vi "UI Main_V1.vi"() -> ()   [LabVIEW 2015]
uses:
  controls/UI Data.ctl
  support/Message Queue/Message Cluster.ctl
  Globals/Global - All UI Loop Stop.vi
  Globals/Global - UI Stream and Variable Connections.vi
  Globals/Global - Configuration Options.vi
  support/User Event - Stop/User Event - Stop.lvlib
  support/Message Queue/Message Queue.lvlib
panel:
  out "Current Logging State":u16(ring) items=["Logging", "Idle (Safe State)"]
  in  "Exit":bool
  out "System Status":string
  in  "Settings Tab":enum32{"UI Commands", "System Monitoring"}(tab)
  in  "Show Live Data":bool
  in  "Live Data Channel":u32 max=7 step=1
  out "Live Data":waveform(dbl)(graph)
  in  "Stop Live Data":bool
  in  "Acquire Live Data":bool
  out "Most recent manually-triggered log file":path
  in  "Force Trigger":bool
  out "Number of Data Files":u32
  out "Actual Loop Period (ticks)":u32
  out "Largest Contiguous Memory (bytes)":dbl(graph)
  out "Resource Utilization (%)":cluster{dbl, "Double":dbl, dbl}(graph)
  out "System Time":timestamp
  out "Connected?":bool
  in  "Connect to Controller":bool
  in  "Controller Address":string
  # "LabVIEW FPGA Waveform Acquisition and Logging on CompactRIO"
  # "Connection Settings"
  # "Live Data"
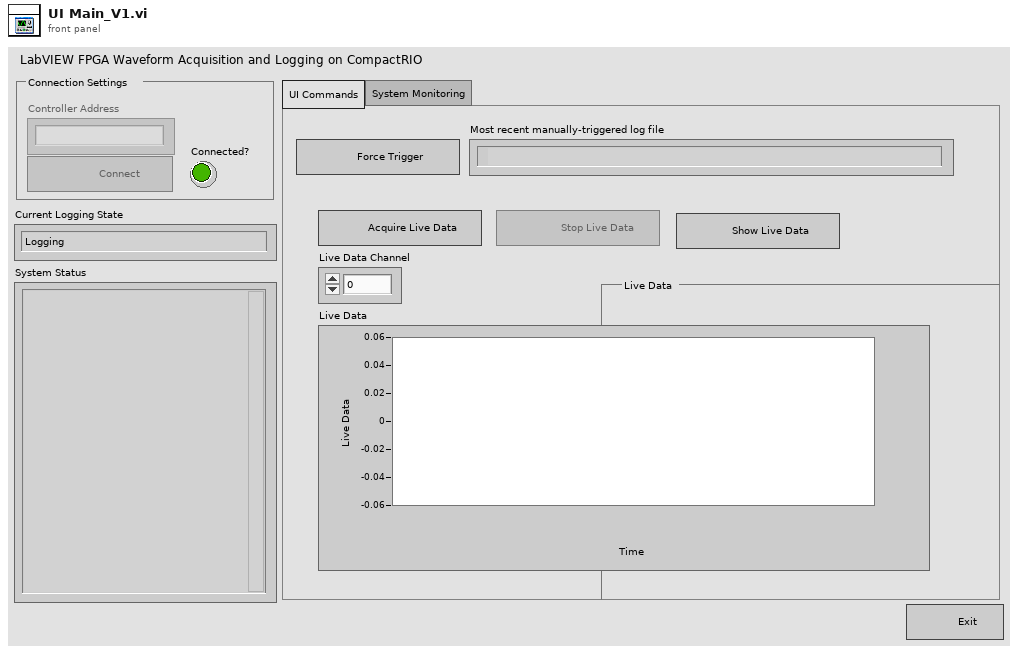
[diagram p1: front panel]
types:
  T1 = typedef "UI Data.ctl" = cluster{"Create Log File Ref":refnum<vi>, "Acquire Live Data Ref":refnum<vi>, "Stop Live Data Ref":refnum<vi>, "Show Live Data Ref":refnum<vi>}
  T2 = typedef "Message Queue.lvlib/All Host Message Queues.ctl" = cluster{"UI":refnum<queue>}
  T3 = typedef "Message Queue.lvlib/Message Cluster.ctl" = cluster{"Message":string, "Message Data":variant}
  T4 = typedef "Variable References.ctl" = cluster{"CPU Usage":refnum<k21>, "Contiguous Memory":refnum<k21>, "Actual Loop Period":refnum<k21>, "Buffer Backlog":refnum<k21>, "Drive Space":refnum<k21>, "Number of Data Files":refnum<k21>, "System Time":refnum<k21>}
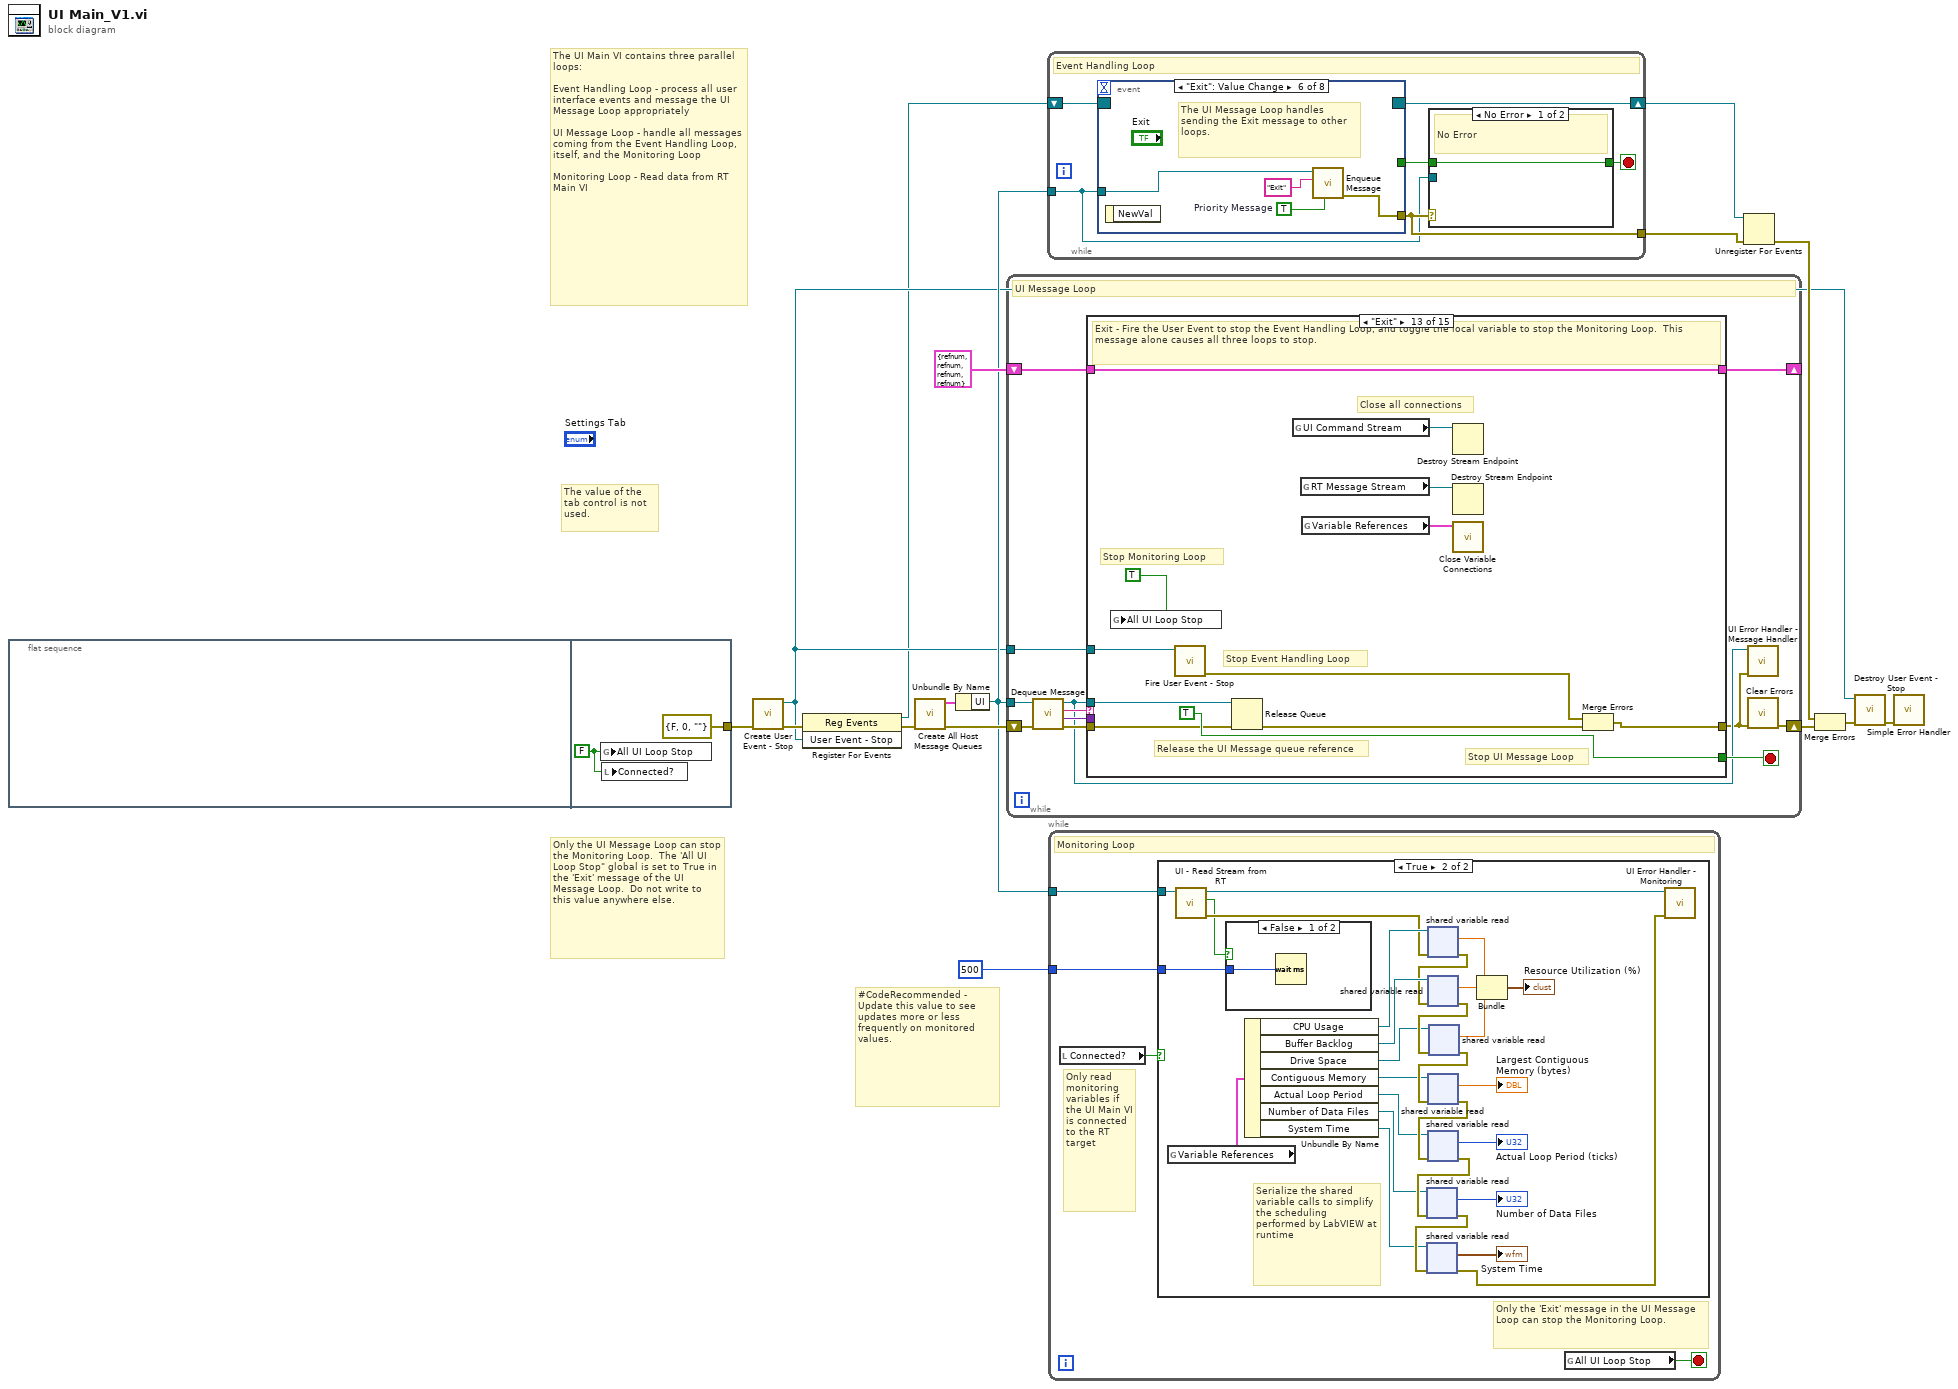
[diagram p0: block diagram]
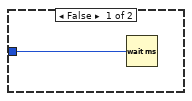
[diagram p2: hidden frame]
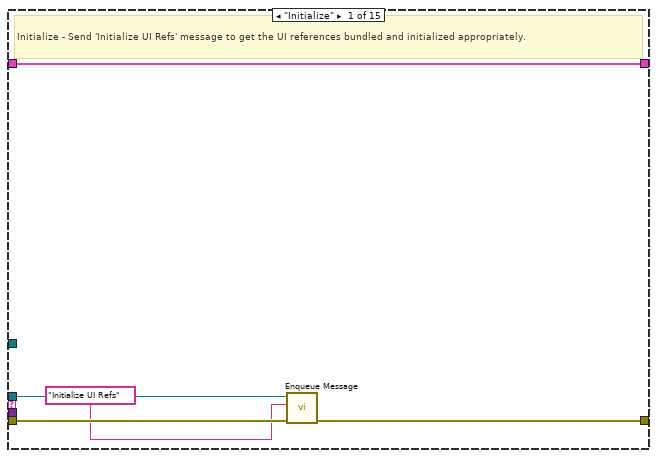
[diagram p4: hidden frame]
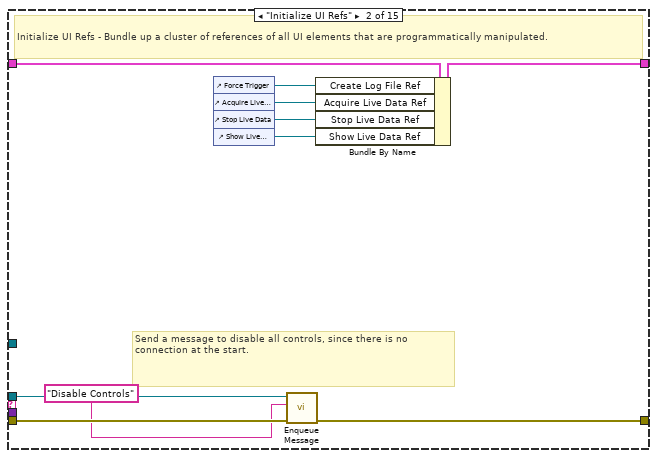
[diagram p5: hidden frame]
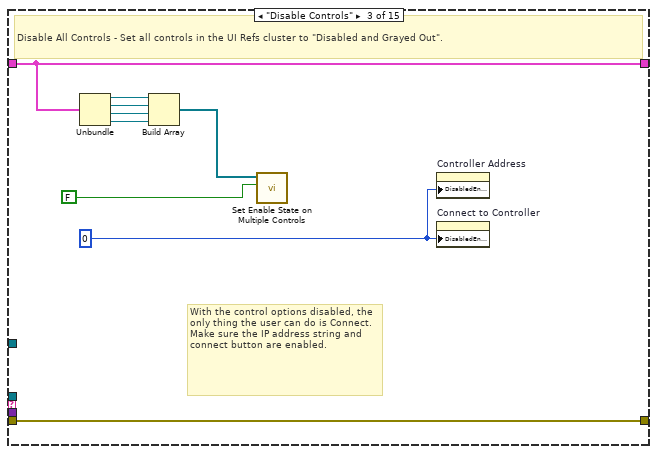
[diagram p6: hidden frame]
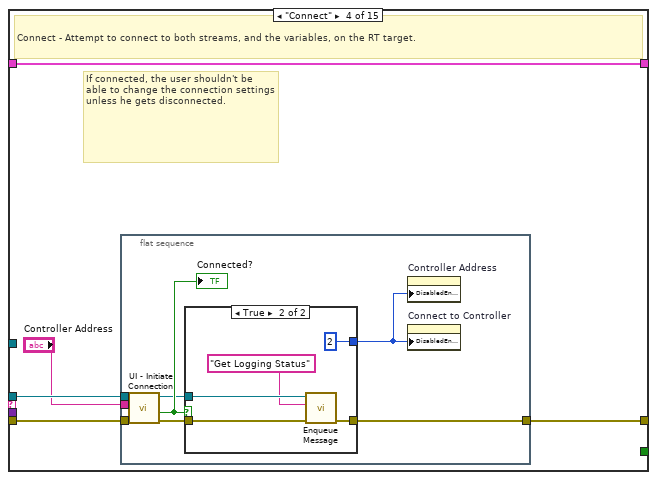
[diagram p7: hidden frame]
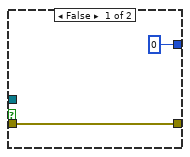
[diagram p8: hidden frame]
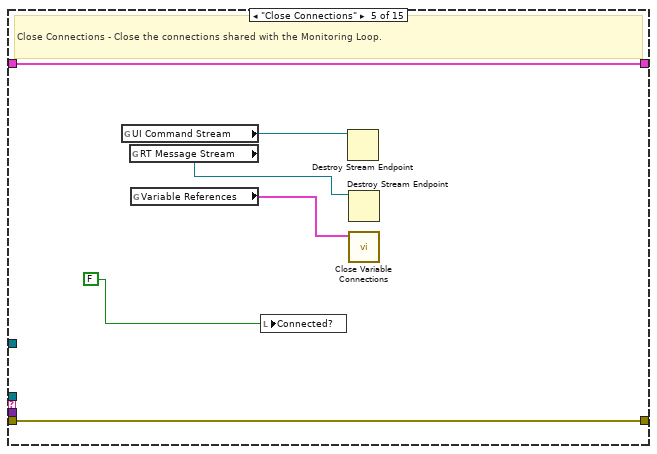
[diagram p9: hidden frame]
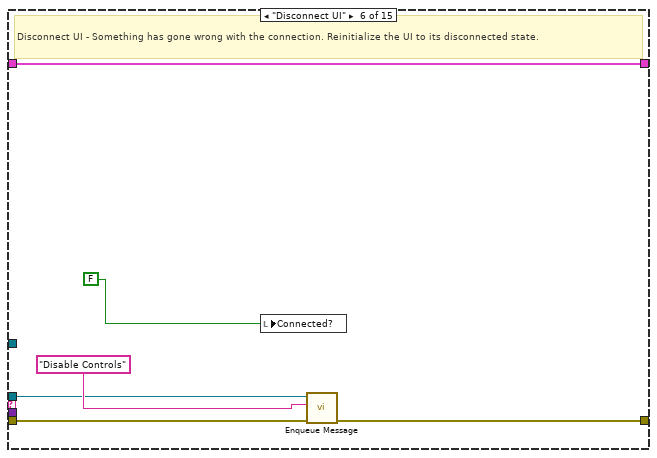
[diagram p10: hidden frame]
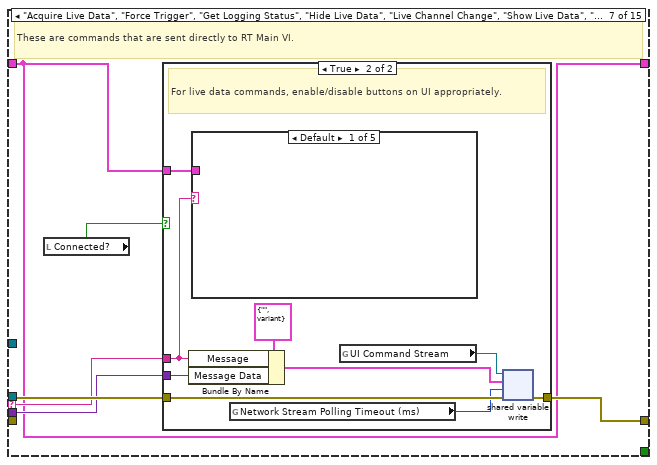
[diagram p11: hidden frame]
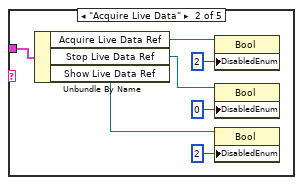
[diagram p13: hidden frame]
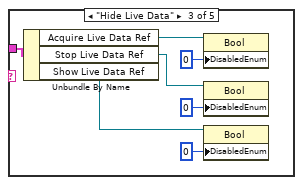
[diagram p14: hidden frame]
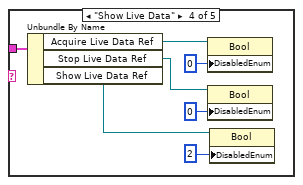
[diagram p15: hidden frame]
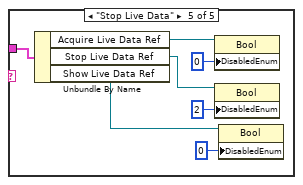
[diagram p16: hidden frame]
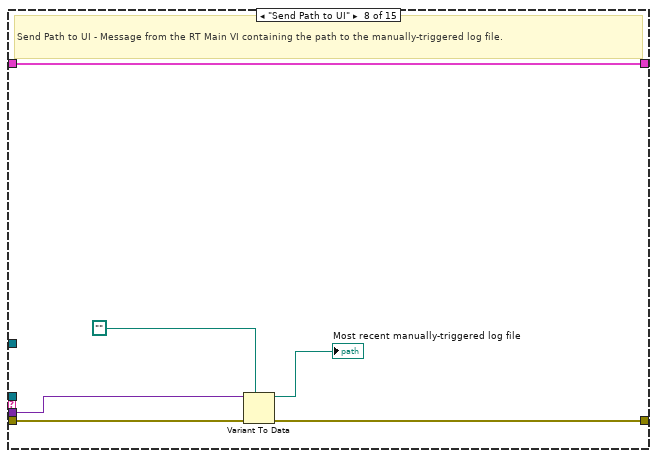
[diagram p17: hidden frame]
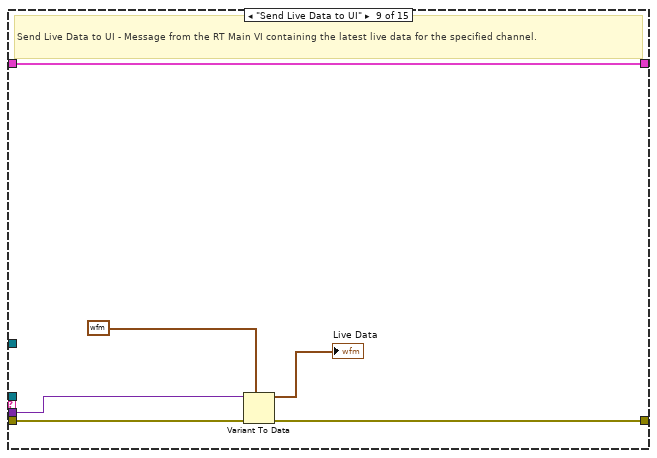
[diagram p18: hidden frame]
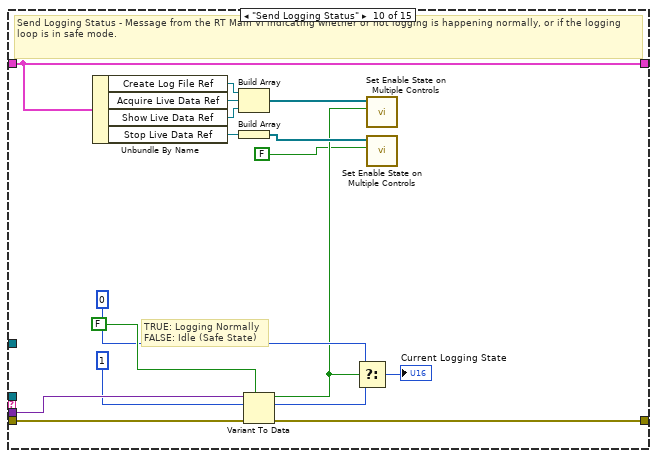
[diagram p19: hidden frame]
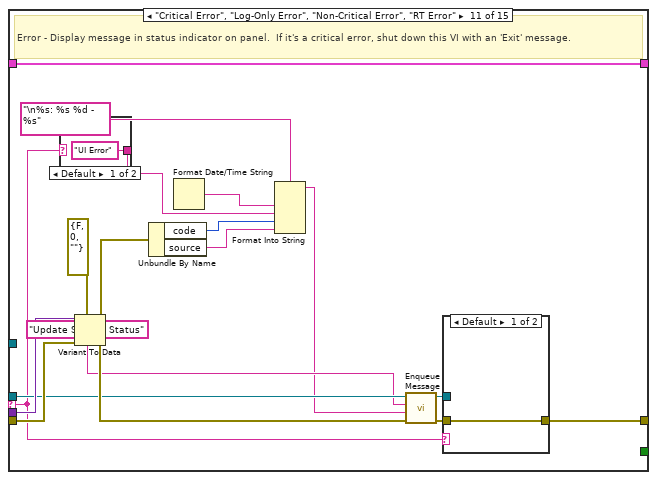
[diagram p20: hidden frame]
diagram:
  # "#CodeRecommended - Update this value to see updates more or less frequently on monitored values."
  # "The UI Main VI contains three parallel loops:\n\nEvent Handling Loop - process all user interface events and message the UI Message Loop appropriately\n\nUI Message Loop - handle all messages coming from the Event Handling Loop, itself, and the Monitoring Loop\n\nMonitoring Loop - Read data from RT Main VI"
  # "The value of the tab control is not used."
  # "Only the UI Message Loop can stop the Monitoring Loop.  The 'All UI Loop Stop\" global is set to True in the 'Exit' message of the UI Message Loop.  Do not write to this value anywhere else."
  n1 = flat-sequence {
    tunnel: [errorcluster {"status"=FALSE, "code"=0, "source"=""} ("error in (no error)")] -> w6
    frame #0 {
    }
    frame #1 {
      w17 = FALSE
      n2 = global write "Global - All UI Loop Stop.vi" "All UI Loop Stop"(w17) -> ()
      n3 = local write "Connected?"(w17) -> ()
    }
  }
  n4 = call "Create User Event - Stop.vi"("error in (no error)"=w6) -> ("error out"=w4:errorcluster, "User Event - Stop"=w2:refnum<user-event>)  [unwired: 9 in]
  n5 = register-events(error in=w4, w2) -> (reference out=w1:refnum<event-registration>, error out=w3:errorcluster)  [unwired: 1 in]
  n6 = call "Create All Host Message Queues.vi"("error in (no error)"=w3) -> ("error out"=w12:errorcluster, "Message Queues out"=w13:T2)  [unwired: 9 in]
  n7 = Unbundle By Name(w13) -> ("UI"=w7:refnum<queue>)
  n8 = while {
    tunnel: w7 -> [w24]
    tunnel: w2 -> [w29]
    shift-right: [w19] -> w16
    shift-left: w12 -> [w28]
    shift-right: [w22] -> _
    shift-left: T1 {"Create Log File Ref"=refnum, "Acquire Live Data Ref"=refnum, "Stop Live Data Ref"=refnum, "Show Live Data Ref"=refnum} ("Measurement UI Controls") -> [w23]
    stop <- w30 stop-if-true
    # "UI Message Loop"
    n9 = call "Dequeue Message.vi"("error in (no error)"=w28, "Message Queue"=w24) -> ("error out"=w27:errorcluster, "Message Data"=w25:variant, "Message"=w26:string, "dup Message Queue"=w21:refnum<queue>)  [unwired: 6 in]
    n10 = case "Message Cases" shown="\"Exit\"" w26 {
      selector: w26 -> [_ _ _ _ _ _ w89 _ _ _ w160 _ _ _ w221]
      tunnel: w21 -> [w32 w41 _ w58 _ w82 _ _ _ _ w164 _ w206 _ _]
      tunnel: w27 -> [w34 w45 w54 w59 w80 w84 w92 w136 w142 w158 w174 w195 w211 w216 _]
      tunnel: [w33 w42 w54 w56 w80 w83 w91 w134 w140 w157 w175 w193 w212 w215 w219] -> w20
      tunnel: [_ _ _ _ _ _ _ _ _ _ _ _ TRUE _ _] -> w30
      tunnel: w25 -> [_ _ _ _ _ _ w90 w133 w139 w156 w172 w192 _ _ _]
      tunnel: w29 -> [_ _ _ _ _ _ _ _ _ _ _ _ w210 _ _]
      tunnel: w23 -> [w35 w44 w53 w57 w79 w86 w88 w135 w141 w151 w176 w194 w208 w214 w217]
      tunnel: [w35 w43 w53 w57 w79 w86 w88 w135 w141 w151 w176 w194 w208 w214 w217] -> w22
      frame "Initialize" {
        # "Initialize - Send 'Initialize UI Refs' message to get the UI references bundled and initialized appropriately."
        n11 = call "Enqueue Message.vi"("error in (no error)"=w34, "Message"="Initialize UI Refs", "Message Queue"=w32) -> ("error out"=w33:errorcluster)  [unwired: 7 in, 1 out]
      }
      frame "Initialize UI Refs" {
        # "Send a message to disable all controls, since there is no connection at the start."
        # "Initialize UI Refs - Bundle up a cluster of references of all UI elements that are programmatically manipulated."
        n12 = control-ref of="Force Trigger"() -> (w39:refnum<vi>)
        n13 = control-ref of="Acquire Live Data"() -> (w38:refnum<vi>)
        n14 = control-ref of="Stop Live Data"() -> (w37:refnum<vi>)
        n15 = control-ref of="Show Live Data"() -> (w36:refnum<vi>)
        n16 = call "Enqueue Message.vi"("error in (no error)"=w45, "Message"="Disable Controls", "Message Queue"=w41) -> ("error out"=w42:errorcluster)  [unwired: 7 in, 1 out]
        n17 = Bundle By Name(cluster=w44, "Create Log File Ref"=w39, "Acquire Live Data Ref"=w38, "Stop Live Data Ref"=w37, "Show Live Data Ref"=w36) -> (w43:T1)
      }
      frame "Disable Controls" {
        w49 = 0
        # "With the control options disabled, the only thing the user can do is Connect. Make sure the IP address string and connect button are enabled."
        # "Disable All Controls - Set all controls in the UI Refs cluster to \"Disabled and Grayed Out\"."
        n18 = Unbundle(w53) -> ("Create Log File Ref"=w52:refnum<vi>, "Acquire Live Data Ref"=w48:refnum<vi>, "Stop Live Data Ref"=w47:refnum<vi>, "Show Live Data Ref"=w46:refnum<vi>)
        n19 = Build Array(w52, w48, w47, w46) -> (w51:refnum<vi>[])
        n20 = call "Set Enable State on Multiple Controls.vi"("Enable?"=FALSE, "Controls"=w51) -> ()  [unwired: 10 in]
        n21 = property on="Controller Address" class="Str"("DisabledEnum"=w49) -> ()  [unwired: 2 in, 2 out]
        n22 = property on="Connect to Controller" class="Bool"("DisabledEnum"=w49) -> ()  [unwired: 2 in, 2 out]
      }
      frame "Connect" {
        # "If connected, the user shouldn't be able to change the connection settings unless he gets disconnected."
        # "Connect - Attempt to connect to both streams, and the variables, on the RT target."
        n23 = flat-sequence {
          tunnel: [w62] -> w56
          tunnel: w59 -> [w67]
          tunnel: w58 -> [w66]
          tunnel: "Controller Address" -> [w65]
          frame #0 {
            n24 = call "UI - Initiate Connection.vi"("error in (no error)"=w67, "Controller Address"=w65, "Message Queue"=w66) -> ("error out"=w64:errorcluster, "Connected?"=w63:bool, "dup Message Queue"=w61:refnum<queue>)  [unwired: 6 in]
            "Connected?" <- w63
            n25 = case shown="True" w63 {
              tunnel: w64 -> [w69 w73]
              tunnel: [w69 w74] -> w62
              tunnel: w61 -> [_ w72]
              tunnel: [0 2] -> w60
              frame False {
              }
              frame True {
                n26 = call "Enqueue Message.vi"("error in (no error)"=w73, "Message"="Get Logging Status", "Message Queue"=w72) -> ("error out"=w74:errorcluster)  [unwired: 7 in, 1 out]
              }
            }
            n27 = property on="Controller Address" class="Str"("DisabledEnum"=w60) -> ()  [unwired: 2 in, 2 out]
            n28 = property on="Connect to Controller" class="Bool"("DisabledEnum"=w60) -> ()  [unwired: 2 in, 2 out]
          }
        }
      }
      frame "Close Connections" {
        # "Close Connections - Close the connections shared with the Monitoring Loop."
        n29 = global read "Global - UI Stream and Variable Connections.vi" "UI Command Stream"() -> (w78:refnum<k21>)
        n30 = global read "Global - UI Stream and Variable Connections.vi" "RT Message Stream"() -> (w77:refnum<k21>)
        n31 = global read "Global - UI Stream and Variable Connections.vi" "Variable References"() -> (w76:T4)
        n32 = local write "Connected?"(FALSE ("Connected?")) -> ()
        n33 = Destroy Stream Endpoint(11:w78) -> ()  [unwired: 1 in, 1 out]
        n34 = Destroy Stream Endpoint(11:w77) -> ()  [unwired: 1 in, 1 out]
        n35 = call "Close Variable Connections.vi"("Variable References"=w76) -> ()  [unwired: 11 in]
      }
      frame "Disconnect UI" {
        # "Disconnect UI - Something has gone wrong with the connection. Reinitialize the UI to its disconnected state."
        n36 = local write "Connected?"(FALSE ("Connected?")) -> ()
        n37 = call "Enqueue Message.vi"("error in (no error)"=w84, "Message"="Disable Controls", "Message Queue"=w82) -> ("error out"=w83:errorcluster)  [unwired: 7 in, 1 out]
      }
      frame "Acquire Live Data", "Force Trigger", "Get Logging Status", "Hide Live Data", "Live Channel Change", "Show Live Data", "Stop Live Data" {
        # "These are commands that are sent directly to RT Main VI."
        n38 = local read "Connected?"() -> (w87:bool)
        n39 = case shown="True" w87 {
          tunnel: w92 -> [w93 w102]
          tunnel: [w93 w101] -> w91
          tunnel: w90 -> [_ w96]
          tunnel: w89 -> [_ w94]
          tunnel: w88 -> [_ w95]
          frame False {
            # "Don't bother trying to send a message to the RT system if UI Main VI isn't even connected"
          }
          frame True {
            # "For live data commands, enable/disable buttons on UI appropriately."
            n40 = Bundle By Name(cluster=T3 {"Message"="", "Message Data"=variant} ("Message Cluster"), "Message"=w94, "Message Data"=w96) -> (w97:T3)
            n41 = case shown="Default" w94 {
              tunnel: w95 -> [_ w109 w110 w119 w130]
              frame Default {
              }
              frame "Acquire Live Data" {
                n42 = Unbundle By Name(w109) -> ("Acquire Live Data Ref"=w108:refnum<vi>, "Stop Live Data Ref"=w107:refnum<vi>, "Show Live Data Ref"=w103:refnum<vi>)
                n43 = property class="Bool"(reference=w108, "DisabledEnum"=u8 2) -> ()  [unwired: 1 in, 2 out]
                n44 = property class="Bool"(reference=w107, "DisabledEnum"=u8 0) -> ()  [unwired: 1 in, 2 out]
                n45 = property class="Bool"(reference=w103, "DisabledEnum"=u8 2) -> ()  [unwired: 1 in, 2 out]
              }
              frame "Hide Live Data" {
                n46 = Unbundle By Name(w110) -> ("Acquire Live Data Ref"=w116:refnum<vi>, "Stop Live Data Ref"=w115:refnum<vi>, "Show Live Data Ref"=w111:refnum<vi>)
                n47 = property class="Bool"(reference=w116, "DisabledEnum"=u8 0) -> ()  [unwired: 1 in, 2 out]
                n48 = property class="Bool"(reference=w115, "DisabledEnum"=u8 0) -> ()  [unwired: 1 in, 2 out]
                n49 = property class="Bool"(reference=w111, "DisabledEnum"=u8 0) -> ()  [unwired: 1 in, 2 out]
              }
              frame "Show Live Data" {
                n50 = Unbundle By Name(w119) -> ("Acquire Live Data Ref"=w123:refnum<vi>, "Stop Live Data Ref"=w122:refnum<vi>, "Show Live Data Ref"=w118:refnum<vi>)
                n51 = property class="Bool"(reference=w123, "DisabledEnum"=u8 0) -> ()  [unwired: 1 in, 2 out]
                n52 = property class="Bool"(reference=w122, "DisabledEnum"=u8 0) -> ()  [unwired: 1 in, 2 out]
                n53 = property class="Bool"(reference=w118, "DisabledEnum"=u8 2) -> ()  [unwired: 1 in, 2 out]
              }
              frame "Stop Live Data" {
                n54 = Unbundle By Name(w130) -> ("Acquire Live Data Ref"=w129:refnum<vi>, "Stop Live Data Ref"=w128:refnum<vi>, "Show Live Data Ref"=w124:refnum<vi>)
                n55 = property class="Bool"(reference=w129, "DisabledEnum"=u8 0) -> ()  [unwired: 1 in, 2 out]
                n56 = property class="Bool"(reference=w128, "DisabledEnum"=u8 2) -> ()  [unwired: 1 in, 2 out]
                n57 = property class="Bool"(reference=w124, "DisabledEnum"=u8 0) -> ()  [unwired: 1 in, 2 out]
              }
            }
            n58 = global read "Global - Configuration Options.vi" "Network Stream Polling Timeout (ms)"() -> (w99:i32)
            n59 = global read "Global - UI Stream and Variable Connections.vi" "UI Command Stream"() -> (w100:refnum<k21>)
            n60 = shared-variable-write(w100, w102, w97, w99) -> (w101:errorcluster)  [unwired: 2 out]
          }
        }
      }
      frame "Send Path to UI" {
        # "Send Path to UI - Message from the RT Main VI containing the path to the manually-triggered log file."
        n61 = Variant To Data(error in=w136, type=path "", Variant=w133) -> (data=→"Most recent manually-triggered log file":path, error out=w134:errorcluster)
      }
      frame "Send Live Data to UI" {
        # "Send Live Data to UI - Message from the RT Main VI containing the latest live data for the specified channel."
        n62 = Variant To Data(error in=w142, type=waveform(dbl) {"t0"=timestamp(0 s since 1904-01-01), "dt"=1.0, "Y"=[]}, Variant=w139) -> (data=→"Live Data":waveform(dbl), error out=w140:errorcluster)
      }
      frame "Send Logging Status" {
        # "TRUE: Logging Normally\nFALSE: Idle (Safe State)"
        # "Send Logging Status - Message from the RT Main VI indicating whether or not logging is happening normally, or if the logging loop is in safe mode."
        n63 = Unbundle By Name(w151) -> ("Create Log File Ref"=w150:refnum<vi>, "Acquire Live Data Ref"=w149:refnum<vi>, "Show Live Data Ref"=w144:refnum<vi>, "Stop Live Data Ref"=w143:refnum<vi>)
        n64 = Build Array(w150, w149, w144) -> (w148:refnum<vi>[])
        n65 = Build Array(w143) -> (w147:refnum<vi>[])
        n66 = Variant To Data(error in=w158, type=FALSE, Variant=w156) -> (data=w146:bool, error out=w157:errorcluster)
        n67 = Select(t=u16 0, s=w146, f=u16 1) -> (s? t:f=→"Current Logging State":u16)
        n68 = call "Set Enable State on Multiple Controls.vi"("Enable?"=w146, "Controls"=w148) -> ()  [unwired: 10 in]
        n69 = call "Set Enable State on Multiple Controls.vi"("Enable?"=FALSE, "Controls"=w147) -> ()  [unwired: 10 in]
      }
      frame "Critical Error", "Log-Only Error", "Non-Critical Error", "RT Error" {
        # "Error - Display message in status indicator on panel.  If it's a critical error, shut down this VI with an 'Exit' message."
        n70 = case shown="Default" w160 {
          selector: w160 -> [_ w183]
          tunnel: ["UI Error" w183] -> w159
          frame Default {
          }
          frame "RT Error" {
          }
        }
        n71 = Variant To Data(error in=w174, type=errorcluster {"status"=FALSE, "code"=0, "source"=""} ("error constant"), Variant=w172) -> (data=w167:errorcluster, error out=w173:errorcluster)
        n72 = Unbundle By Name(w167) -> ("code"=w166:i32, "source"=w170:string)
        n73 = Format Date/Time String() -> (date/time string=w169:string)  [unwired: 3 in]
        n74 = Format Into String(format string="\n%s: %s %d - %s", w169, w159, w166, w170) -> (resulting string=w161:string)  [unwired: 2 in, 1 out]
        n75 = call "Enqueue Message.vi"("error in (no error)"=w173, "Message Data"=w161, "Message"="Update System Status", "Message Queue"=w164) -> ("error out"=w165:errorcluster, "dup Message Queue"=w163:refnum<queue>)  [unwired: 6 in]
        n76 = case shown="Default" w160 {
          tunnel: w165 -> [w177 w181]
          tunnel: w163 -> [_ w179]
          tunnel: [w177 w180] -> w175
          frame Default {
          }
          frame "Critical Error" {
            n77 = call "Enqueue Message.vi"("error in (no error)"=w181, "Message"="Exit", "Message Queue"=w179) -> ("error out"=w180:errorcluster)  [unwired: 7 in, 1 out]
          }
        }
      }
      frame "Update System Status" {
        # "#CodeRecommended - The code below ensures that the System Status string value does not become too large.  It uses the same maximum size as the RT error log to determine whether or not to remove the last half of the log string. Change this logic if you wish to maintain more/less of the information in the System Status string."
        # "Update System Status - Add a new string to the beginning of the System Status string on the UI."
        n78 = Variant To Data(error in=w195, type="", Variant=w192) -> (data=w189:string, error out=w193:errorcluster)
        n79 = global read "Global - Configuration Options.vi" "Error Log Max Size (bytes)"() -> (w185:i64)
        n80 = local read "System Status"() -> (w187:string)
        n81 = String Length(string=w187) -> (length=w188:i32)
        n82 = Greater?(x=w188, y=w185) -> (0:w186:bool)
        n83 = case shown="True" w186 {
          tunnel: w187 -> [w196 w200]
          tunnel: w185 -> [_ w199]
          tunnel: [w196 w201] -> w184
          frame False {
          }
          frame True {
            n84 = Divide(x=w199, y=i64 2) -> (x/y=w198:dbl)
            n85 = String Subset(string=w200, length (rest)=w198) -> (substring=w201:string)  [unwired: 1 in]
          }
        }
        n86 = Concatenate Strings(w189, w184) -> (→"System Status":string)
      }
      frame "Exit" {
        # "Close all connections"
        # "Stop Monitoring Loop"
        # "Stop Event Handling Loop"
        # "Release the UI Message queue reference"
        # "Stop UI Message Loop"
        # "Exit - Fire the User Event to stop the Event Handling Loop, and toggle the local variable to stop the Monitoring Loop.  This message alone causes all three loops to stop."
        n87 = global write "Global - All UI Loop Stop.vi" "All UI Loop Stop"(TRUE ("Stop Monitoring Loop")) -> ()
        n88 = call "Fire User Event - Stop.vi"("User Event - Stop"=w210) -> ("error out"=w209:errorcluster)  [unwired: 10 in]
        n89 = Release Queue(queue=w206, error in (no error)=w211) -> (error out=w207:errorcluster)  [unwired: 1 in, 2 out]
        n90 = global read "Global - UI Stream and Variable Connections.vi" "UI Command Stream"() -> (w204:refnum<k21>)
        n91 = global read "Global - UI Stream and Variable Connections.vi" "RT Message Stream"() -> (w203:refnum<k21>)
        n92 = global read "Global - UI Stream and Variable Connections.vi" "Variable References"() -> (w202:T4)
        n93 = Destroy Stream Endpoint(11:w204) -> ()  [unwired: 1 in, 1 out]
        n94 = Destroy Stream Endpoint(11:w203) -> ()  [unwired: 1 in, 1 out]
        n95 = call "Close Variable Connections.vi"("Variable References"=w202) -> ()  [unwired: 11 in]
        n96 = Merge Errors(w209, w207) -> (w212:errorcluster)
      }
      frame "---Copy This Frame---" {
        # "Duplicate this frame when creating new messages.  Change this comment in the duplicated frame to describe this message."
        n97 = Merge Errors(w216) -> (w215:errorcluster)
      }
      frame Default {
        # "'Default' case only runs if there is a message that isn't defined in any of the other cases.  Output a programming error."
        n98 = Format Into String(format string="The invalid message string \"%s\" was received in the Message Handling Loop." ("Invalid Message Loop Message"), w221) -> (resulting string=w218:string)  [unwired: 2 in, 1 out]
        n99 = call <vilib>:"Error Cluster From Error Code.vi"("error message (\"\")"=w218, "error code (0)"=1) -> ("error out"=w219:errorcluster)  [unwired: 7 in]
      }
    }
    n100 = call "UI Error Handler - Message Handler.vi"("error in (no error)"=w20, "Message Queue"=w21) -> ()  [unwired: 9 in, 1 out]
    n101 = call <vilib>:"Clear Errors.vi"("error in (no error)"=w20) -> ("error out"=w19:errorcluster)  [unwired: 5 in, 1 out]
  }
  n102 = while {
    tunnel: w7 -> [w224]
    tunnel: [w226] -> w15
    shift-right: [w223] -> w10
    shift-left: w1 -> [w225]
    stop <- w227 stop-if-true
    # "Event Handling Loop"
    n103 = event shown="[5] \"Exit\": Value Change" {
      selector: w225 -> [_ _ _ _ _ _ _ _]
      dyn-events: [_ _ _ _ _ _ _ _] -> w223
      timeout: _ -> [_ _ _ _ _ _ _ _]
      tunnel: [_ _ _ _ _ _ TRUE ("Discard?") _] -> w228
      tunnel: w224 -> [w234 w237 w240 w243 w247 w250 _ w260]
      tunnel: [w236 w239 w242 w245 w249 w253 _ w259] -> w226
      event "Connect to Controller": Value Change {
        n104 = event-data() -> ()  [unwired: 1 in, 1 out]
        n105 = call "Enqueue Message.vi"("Message"="Connect", "Message Queue"=w234) -> ("error out"=w236:errorcluster)  [unwired: 8 in, 1 out]
      }
      event "Force Trigger": Value Change {
        n106 = event-data() -> ()  [unwired: 1 in, 1 out]
        n107 = call "Enqueue Message.vi"("Message"="Force Trigger", "Message Queue"=w237) -> ("error out"=w239:errorcluster)  [unwired: 8 in, 1 out]
      }
      event "Acquire Live Data": Value Change {
        n108 = event-data() -> ()  [unwired: 1 in, 1 out]
        n109 = call "Enqueue Message.vi"("Message"="Acquire Live Data", "Message Queue"=w240) -> ("error out"=w242:errorcluster)  [unwired: 8 in, 1 out]
      }
      event "Stop Live Data": Value Change {
        n110 = event-data() -> ()  [unwired: 1 in, 1 out]
        n111 = call "Enqueue Message.vi"("Message"="Stop Live Data", "Message Queue"=w243) -> ("error out"=w245:errorcluster)  [unwired: 8 in, 1 out]
      }
      event "Live Data Channel": Value Change {
        n112 = event-data() -> ()  [unwired: 1 in, 1 out]
        n113 = call "Enqueue Message.vi"("Message Data"="Live Data Channel", "Message"="Live Channel Change", "Message Queue"=w247) -> ("error out"=w249:errorcluster)  [unwired: 7 in, 1 out]
      }
      event "Exit": Value Change {
        w251 = TRUE  # Priority Message
        # "The UI Message Loop handles sending the Exit message to other loops."
        n114 = event-data() -> ()  [unwired: 1 in, 1 out]
        n115 = call "Enqueue Message.vi"("Priority Message? (F)"=w251, "Message"="Exit", "Message Queue"=w250) -> ("error out"=w253:errorcluster)  [unwired: 7 in, 1 out]
      }
      event User Event {
        # "The Message Handling Loop processed an \"Exit\" message, which fired this event to stop the Event Handling Loop."
        n116 = event-data() -> ()  [unwired: 1 in, 1 out]
      }
      event "Show Live Data": Value Change {
        n117 = event-data() -> ()  [unwired: 1 in, 1 out]
        n118 = Select(t="Show Live Data" ("Message"), s="Show Live Data", f="Hide Live Data" ("Message")) -> (s? t:f=w255:string)
        n119 = call "Enqueue Message.vi"("Message"=w255, "Message Queue"=w260) -> ("error out"=w259:errorcluster)  [unwired: 8 in, 1 out]
      }
    }
    n120 = case shown="No Error" w226 {
      tunnel: [w229 TRUE ("Discard?")] -> w227
      tunnel: w228 -> [w229 _]
      tunnel: w224 -> [_ w230]
      frame No Error {
        # "No Error"
      }
      frame Error {
        # "On error, send Exit message, and stop loop."
        n121 = call "Enqueue Message.vi"("Priority Message? (F)"=TRUE ("Discard?"), "Message"="Exit", "Message Queue"=w230) -> ()  [unwired: 7 in, 2 out]
      }
    }
  }
  n122 = while {
    tunnel: w7 -> [w263]
    tunnel: u32 500 ("milliseconds to wait") -> [w261]
    stop <- w264 stop-if-true
    # "Only read monitoring variables if the UI Main VI is connected to the RT target"
    # "Only the 'Exit' message in the UI Message Loop can stop the Monitoring Loop."
    # "Monitoring Loop"
    n123 = local read "Connected?"() -> (w262:bool)
    n124 = case shown="True" w262 {
      tunnel: w263 -> [_ w289]
      tunnel: w261 -> [w265 w266]
      frame False {
        n125 = Wait (ms)(milliseconds to wait=w265) -> ()  [unwired: 1 out]
      }
      frame True {
        # "Serialize the shared variable calls to simplify the scheduling performed by LabVIEW at runtime"
        n126 = global read "Global - UI Stream and Variable Connections.vi" "Variable References"() -> (w287:T4)
        n127 = call "UI - Read Stream from RT.vi"("Message Queue"=w289) -> ("error out"=w290:errorcluster, "Message Received?"=w267:bool, "dup Message Queue"=w288:refnum<queue>)  [unwired: 8 in]
        n128 = case shown="False" w267 {
          tunnel: w266 -> [w294 _]
          frame False {
            n129 = Wait (ms)(milliseconds to wait=w294) -> ()  [unwired: 1 out]
          }
          frame True {
            # "If a message was received, immediately read again"
          }
        }
        n130 = Unbundle By Name(w287) -> ("CPU Usage"=w292:refnum<k21>, "Buffer Backlog"=w291:refnum<k21>, "Drive Space"=w268:refnum<k21>, "Contiguous Memory"=w279:refnum<k21>, "Actual Loop Period"=w276:refnum<k21>, "Number of Data Files"=w273:refnum<k21>, "System Time"=w269:refnum<k21>)
        n131 = shared-variable-read(w292, w290) -> (w286:errorcluster, w284:dbl)  [unwired: 2 out]
        n132 = shared-variable-read(w291, w286) -> (w285:errorcluster, w283:dbl)  [unwired: 2 out]
        n133 = shared-variable-read(w268, w285) -> (w280:errorcluster, w282:dbl)  [unwired: 2 out]
        n134 = shared-variable-read(w279, w280) -> (w277:errorcluster, →"Largest Contiguous Memory (bytes)":dbl)  [unwired: 2 out]
        n135 = shared-variable-read(w276, w277) -> (w275:errorcluster, →"Actual Loop Period (ticks)":u32)  [unwired: 2 out]
        n136 = shared-variable-read(w273, w275) -> (w272:errorcluster, →"Number of Data Files":u32)  [unwired: 2 out]
        n137 = shared-variable-read(w269, w272) -> (w270:errorcluster, →"System Time":timestamp)  [unwired: 2 out]
        n138 = Bundle(w284, "Double"=w283, w282) -> (→"Resource Utilization (%)":cluster{dbl, "Double":dbl, dbl})  [unwired: 1 in]
        n139 = call "UI Error Handler - Monitoring.vi"("error in (no error)"=w270, "Message Queue"=w288) -> ()  [unwired: 9 in, 1 out]
      }
    }
    n140 = global read "Global - All UI Loop Stop.vi" "All UI Loop Stop"() -> (w264:bool)
  }
  n141 = Unregister For Events(event registration refnum=w10, error in=w15) -> (error out=w11:errorcluster)
  n142 = Merge Errors(w11, w16) -> (w14:errorcluster)
  n143 = call "Destroy User Event - Stop.vi"("error in (no error)"=w14, "User Event - Stop"=w2) -> ("error out"=w8:errorcluster)  [unwired: 9 in]
  n144 = call <vilib>:"Simple Error Handler.vi"("error in (no error)"=w8) -> ()  [unwired: 4 in, 5 out]
